vi "sessionOfTrials.vi"() -> ()   [LabVIEW 2017]
uses:
  <vilib>/Utility/file.llb/Read Delimited Spreadsheet (DBL).vi
  <vilib>/Utility/file.llb/Write Delimited Spreadsheet (I64).vi
panel:
  in  "Choice/goal platforms up or down?":string(combo)
  in  "Rat ID":string
  out "choices":i32[][](array[numeric])
  in  "Goal \nplatform":i32
  in  "start platform":i32
  in  "Number of trials to run":i32
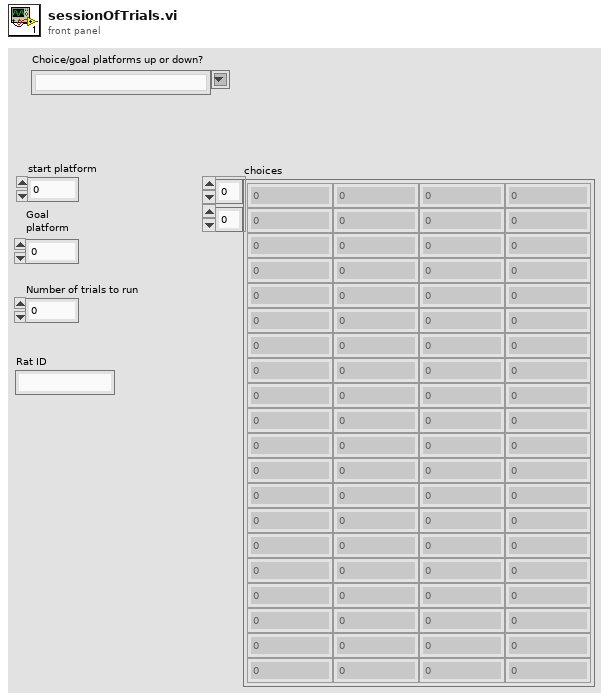
[diagram p1: front panel]
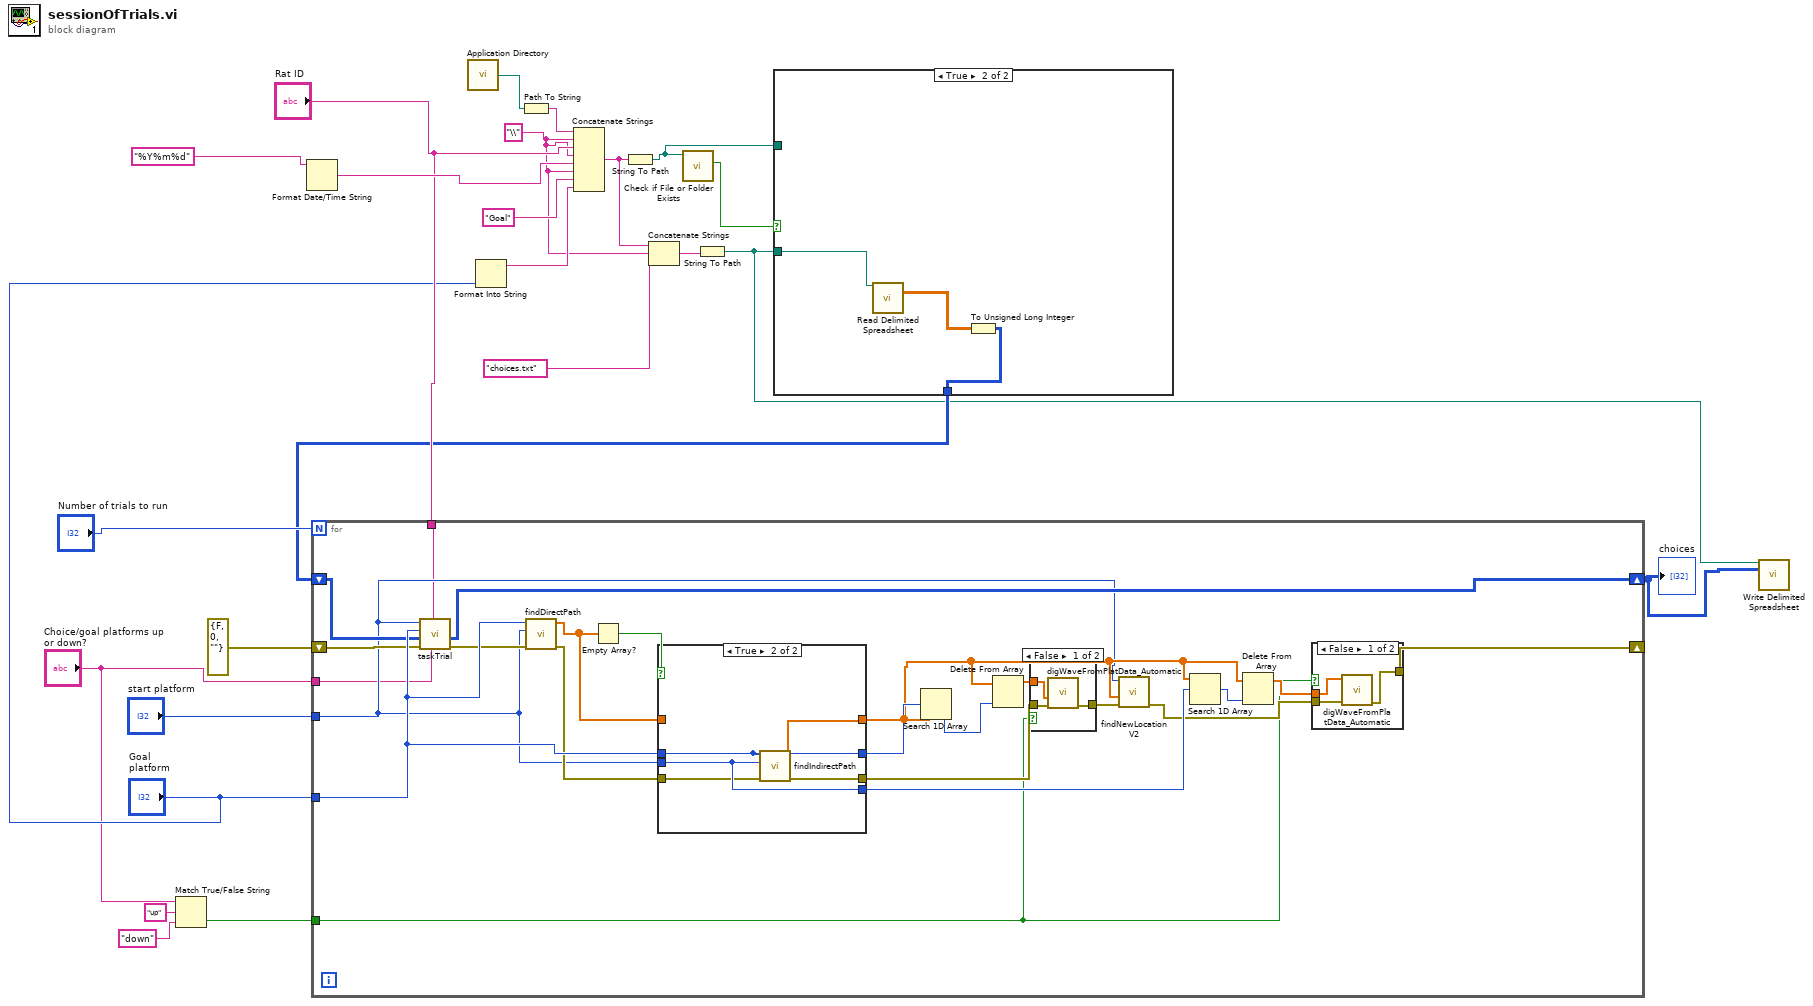
[diagram p0: block diagram]
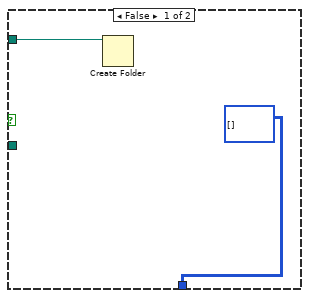
[diagram p2: hidden frame]
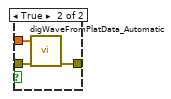
[diagram p3: hidden frame]
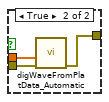
[diagram p4: hidden frame]
diagram:
  w11 = "\\" ("string")
  n1 = Match True/False String(2:"down" ("false string"), 3:"up" ("true string"), 4:"Choice/goal platforms up or down?") -> (0:w1:bool)  [unwired: 1 out]
  n2 = Format Date/Time String(time format string (%c)="%Y%m%d" ("time string")) -> (date/time string=w19:string)  [unwired: 2 in]
  n3 = call <vilib>:"Application Directory.vi"() -> ("Application Directory"=w18:path)
  n4 = Format Into String("Goal \nplatform") -> (resulting string=w13:string)  [unwired: 3 in, 1 out]
  n5 = Path To String(path=w18) -> (string=w21:string)
  n6 = Concatenate Strings(w21, w11, "Rat ID", w11, w19, w11, "Goal" ("string"), w13) -> (w10:string)
  n7 = String To Path(string=w10) -> (path=w6:path)
  n8 = Concatenate Strings(w10, w11, "choices.txt" ("string")) -> (w8:string)
  n9 = call <vilib>:"Check if File or Folder Exists.vi"("path"=w6) -> ("file or folder exists?"=w12:bool)  [unwired: 8 in, 2 out]
  n10 = String To Path(string=w8) -> (path=w5:path)
  n11 = case shown="True" w12 {
    tunnel: w5 -> [_ w29]
    tunnel: [i32[][] [] ("previousChoices") w27] -> w7
    tunnel: w6 -> [w25 _]
    frame False {
      n12 = Create Folder(path (use dialog)=w25) -> ()  [unwired: 2 in, 3 out]
    }
    frame True {
      n13 = call-poly <vilib>:"Read Delimited Spreadsheet.vi"("file path (dialog if empty)"=w29) -> ("all rows"=w28:dbl[][])  [unwired: 9 in, 5 out]
      n14 = To Unsigned Long Integer(number=w28) -> (unsigned 32bit integer=w27:u32[][])
    }
  }
  n15 = for {
    N: "Number of trials to run" -> [_]
    tunnel: "Goal \nplatform" -> [w51]
    tunnel: "start platform" -> [w34]
    shift-right: [w37] -> _
    shift-left: errorcluster {"status"=FALSE, "code"=0, "source"=""} ("error in (no error)") -> [w38]
    shift-right: [w35] -> w17
    shift-left: w7 -> [w36]
    tunnel: "Rat ID" -> [w32]
    tunnel: "Choice/goal platforms up or down?" -> [w31]
    tunnel: w1 -> [w30]
    n16 = call "taskTrial.vi"("up or down"=w31, "Rat ID"=w32, "error in (no error)"=w38, "previousChoices"=w36, "Goal \nplatform"=w51, "Start \nplatform"=w34) -> ("error out"=w41:errorcluster, "previousChoices updated"=w35:i32[][])  [unwired: 3 in, 1 out]
    n17 = call "findDirectPath.vi"("error in (no error)"=w41, "goal platform"=w34, "start platform"=w51) -> ("error out"=w40:errorcluster, "path"=w50:dbl[])  [unwired: 6 in, 1 out]
    n18 = Empty Array?(array=w50) -> (empty?=w52:bool)
    n19 = case shown="True" w52 {
      tunnel: w34 -> [w66 w71]
      tunnel: w51 -> [w67 w72]
      tunnel: w50 -> [w68 _]
      tunnel: [w68 w73] -> w44
      tunnel: [w67 w72] -> w49
      tunnel: [w66 w71] -> w46
      tunnel: w40 -> [w65 w70]
      tunnel: [w65 w69] -> w39
      frame False {
      }
      frame True {
        n20 = call "findIndirectPath.vi"("error in (no error)"=w70, "goal platform"=w71, "start platform"=w72) -> ("error out"=w69:errorcluster, "path between start and goal"=w73:dbl[])  [unwired: 3 in, 4 out]
      }
    }
    n21 = Search 1D Array(1D array=w44, element=w49) -> (index of element=w33:i32)  [unwired: 1 in]
    n22 = Delete From Array(array=w44, index=w33) -> (array with subset deleted=w48:dbl[])  [unwired: 1 in, 1 out]
    n23 = case shown="False" w30 {
      tunnel: w48 -> [w53 w58]
      tunnel: [w54 w57] -> w47
      tunnel: w39 -> [w55 w56]
      frame False {
        n24 = call "digWaveFromPlatData_Automatic.vi"("error in (no error)"=w55, "Platforms\nto lower"=w53) -> ("error out"=w54:errorcluster)  [unwired: 9 in]
      }
      frame True {
        n25 = call "digWaveFromPlatData_Automatic.vi"("error in (no error)"=w56, "Platforms\nto raise"=w58) -> ("error out"=w57:errorcluster)  [unwired: 9 in]
      }
    }
    n26 = call "findNewLocationV2.vi"("error in (no error)"=w47, "possible \nlocations"=w44, "goal location"=w34) -> ("error out"=w42:errorcluster)  [unwired: 7 in, 1 out]
    n27 = Search 1D Array(1D array=w44, element=w46) -> (index of element=w45:i32)  [unwired: 1 in]
    n28 = Delete From Array(array=w44, index=w45) -> (array with subset deleted=w43:dbl[])  [unwired: 1 in, 1 out]
    n29 = case shown="False" w30 {
      tunnel: w43 -> [w61 w64]
      tunnel: w42 -> [w60 w63]
      tunnel: [w59 w62] -> w37
      frame False {
        n30 = call "digWaveFromPlatData_Automatic.vi"("error in (no error)"=w60, "Platforms\nto raise"=w61) -> ("error out"=w59:errorcluster)  [unwired: 9 in]
      }
      frame True {
        n31 = call "digWaveFromPlatData_Automatic.vi"("error in (no error)"=w63, "Platforms\nto lower"=w64) -> ("error out"=w62:errorcluster)  [unwired: 9 in]
      }
    }
  }
  "choices" <- w17
  n32 = call-poly <vilib>:"Write Delimited Spreadsheet.vi"("file path (dialog if empty)"=w5, "2D data"=w17) -> ()  [unwired: 12 in, 2 out]
